vi "Test Variant to String.vi"() -> ()   [LabVIEW 2019, in "LV-Data.lvclass"]
uses:
  LV-Data.lvclass
panel:
  out "error out 2":errorcluster
  out "Value":string
  in  "1D Array":dbl[](array[numeric])
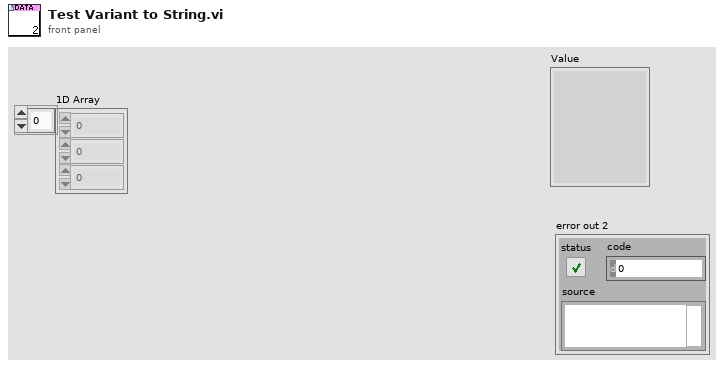
[diagram p1: front panel]
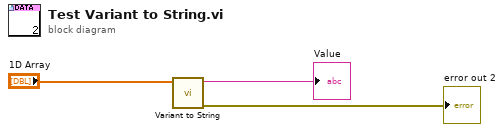
[diagram p0: block diagram]
diagram:
  n1 = call "Variant to String.vi"("Data (Variant)"="1D Array") -> ("error out"=→"error out 2":errorcluster, "String"=→"Value":string)  [unwired: 9 in]
